vi "Assemble Main ViewManager.vi"(8 "Stop Process View":refnum<class "Stop Process View Definition.lvclass">, 9 "Entry Console View":refnum<class "Entry Console View Definition.lvclass">, 10 "Car Position Simulation View":refnum<class "Car Position Simulation View Definition.lvclass">, 11 "Car Wash Display ViewManager":refnum<class "Car Wash Display ViewManager.lvclass">) -> (3 "Main ViewManager out":refnum<class "Main ViewManager.lvclass">)   [LabVIEW 2019, in "Main ViewManager.lvclass"]
uses:
  <vilib>/gpm_packages/@cs/Car-wash/Source/Main ViewManager/Main ViewManager/Main ViewManager.lvclass
  <vilib>/gpm_packages/@cs/mva-viewable/Source/IViewManager/IViewManager/IViewManager.lvclass
  <vilib>/gpm_packages/@cs/Car-wash/Source/Entry Console View Definition/Entry Console View Definition/Entry Console View Definition.lvclass
  C:/Program Files/National Instruments/LabVIEW 2019/vi.lib/gpm_packages/@cs/mva-viewable/Source/IViewable/IViewable/IViewable.lvclass
  C:/Program Files/National Instruments/LabVIEW 2019/vi.lib/gpm_packages/@cs/mva-viewable/Source/ActorEvents/IEventAggregator/IEventAggregator.lvclass
  C:/Program Files/National Instruments/LabVIEW 2019/vi.lib/gpm_packages/@cs/mva-core/Source/IObserver/IObserver/IObserver.lvclass
  C:/Program Files/National Instruments/LabVIEW 2019/vi.lib/ActorFramework/Actor/Actor.lvclass
  <vilib>/gpm_packages/@cs/Car-wash/Source/Car Wash Display ViewManager/Car Wash Display ViewManager/Car Wash Display ViewManager.lvclass
  C:/Program Files/National Instruments/LabVIEW 2019/vi.lib/gpm_packages/@cs/mva-viewable/Source/IViewManager/IViewManager/IViewManager.lvclass
  <vilib>/gpm_packages/@cs/Car-wash/Source/Car Position Simulation View Definition/Car Position Simulation View Definition/Car Position Simulation View Definition.lvclass
  <vilib>/gpm_packages/@cs/Car-wash/Source/Stop Process View Definition/Stop Process View Definition.lvclass
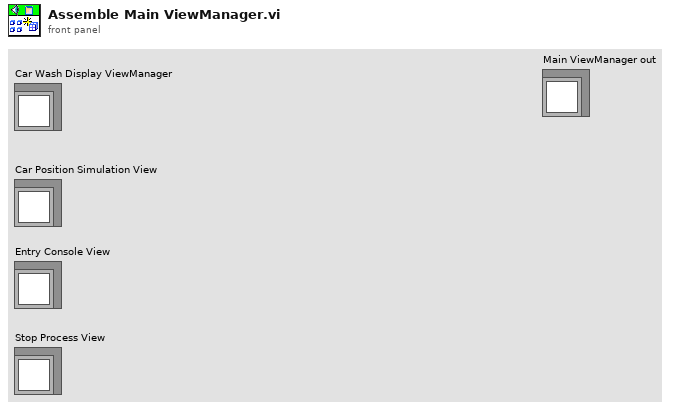
[diagram p1: front panel]
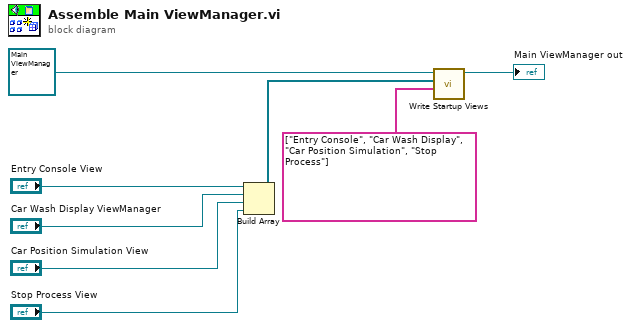
[diagram p0: block diagram]
diagram:
  n1 = Build Array("Entry Console View", "Car Wash Display ViewManager", "Car Position Simulation View", "Stop Process View") -> (w6:refnum<class "IViewable.lvclass">[])
  n2 = call <vilib>:"Write Startup Views.vi"("View Labels"=string[] ["Entry Console", "Car Wash Display", "Car Position Simulation", "Stop Process"], "Startup Views"=w6, "IViewManager in"=refnum<class "Main ViewManager.lvclass"> refnum ("Main ViewManager.lvlib:Main ViewManager.lvclass")) -> ("IViewManager out"=→"Main ViewManager out":refnum<class "Main ViewManager.lvclass">)  [unwired: 8 in]
